vi "glb_data.vi"() -> ()   [LabVIEW 2014]
panel:
  in  "冷却系统模块":T1(array[cluster])
  in  "冷却系统模块值":string[](array[string])
  in  "FPGA模块值":string[](array[string])
  in  "主界面配置类":T2={"侧边栏数据"=[], "界面刷间隔率"=1000.0}
  in  "show配置":T3
  in  "测试模块值8":string[](array[string])
  in  "测试模块值7":string[](array[string])
  in  "测试模块值6":string[](array[string])
  in  "测试模块值5":string[](array[string])
  in  "测试模块值4":string[](array[string])
  in  "测试模块值3":string[](array[string])
  in  "测试模块值2":string[](array[string])
  in  "测试模块值1":string[](array[string])
  in  "cRIO模块值":string[](array[string])
  in  "GPS模块值":string[](array[string])
  in  "OBD模块值":string[](array[string])
  in  "cRIO模块":T1(array[cluster])
  in  "测试模块8":T1(array[cluster])
  in  "测试模块7":T1(array[cluster])
  in  "测试模块6":T1(array[cluster])
  in  "测试模块5":T1(array[cluster])
  in  "测试模块4":T1(array[cluster])
  in  "测试模块3":T1(array[cluster])
  in  "测试模块2":T1(array[cluster])
  in  "测试模块1":T1(array[cluster])
  in  "GPS模块":T1(array[cluster])
  in  "OBD模块":T1(array[cluster])
  in  "数据属性":T4
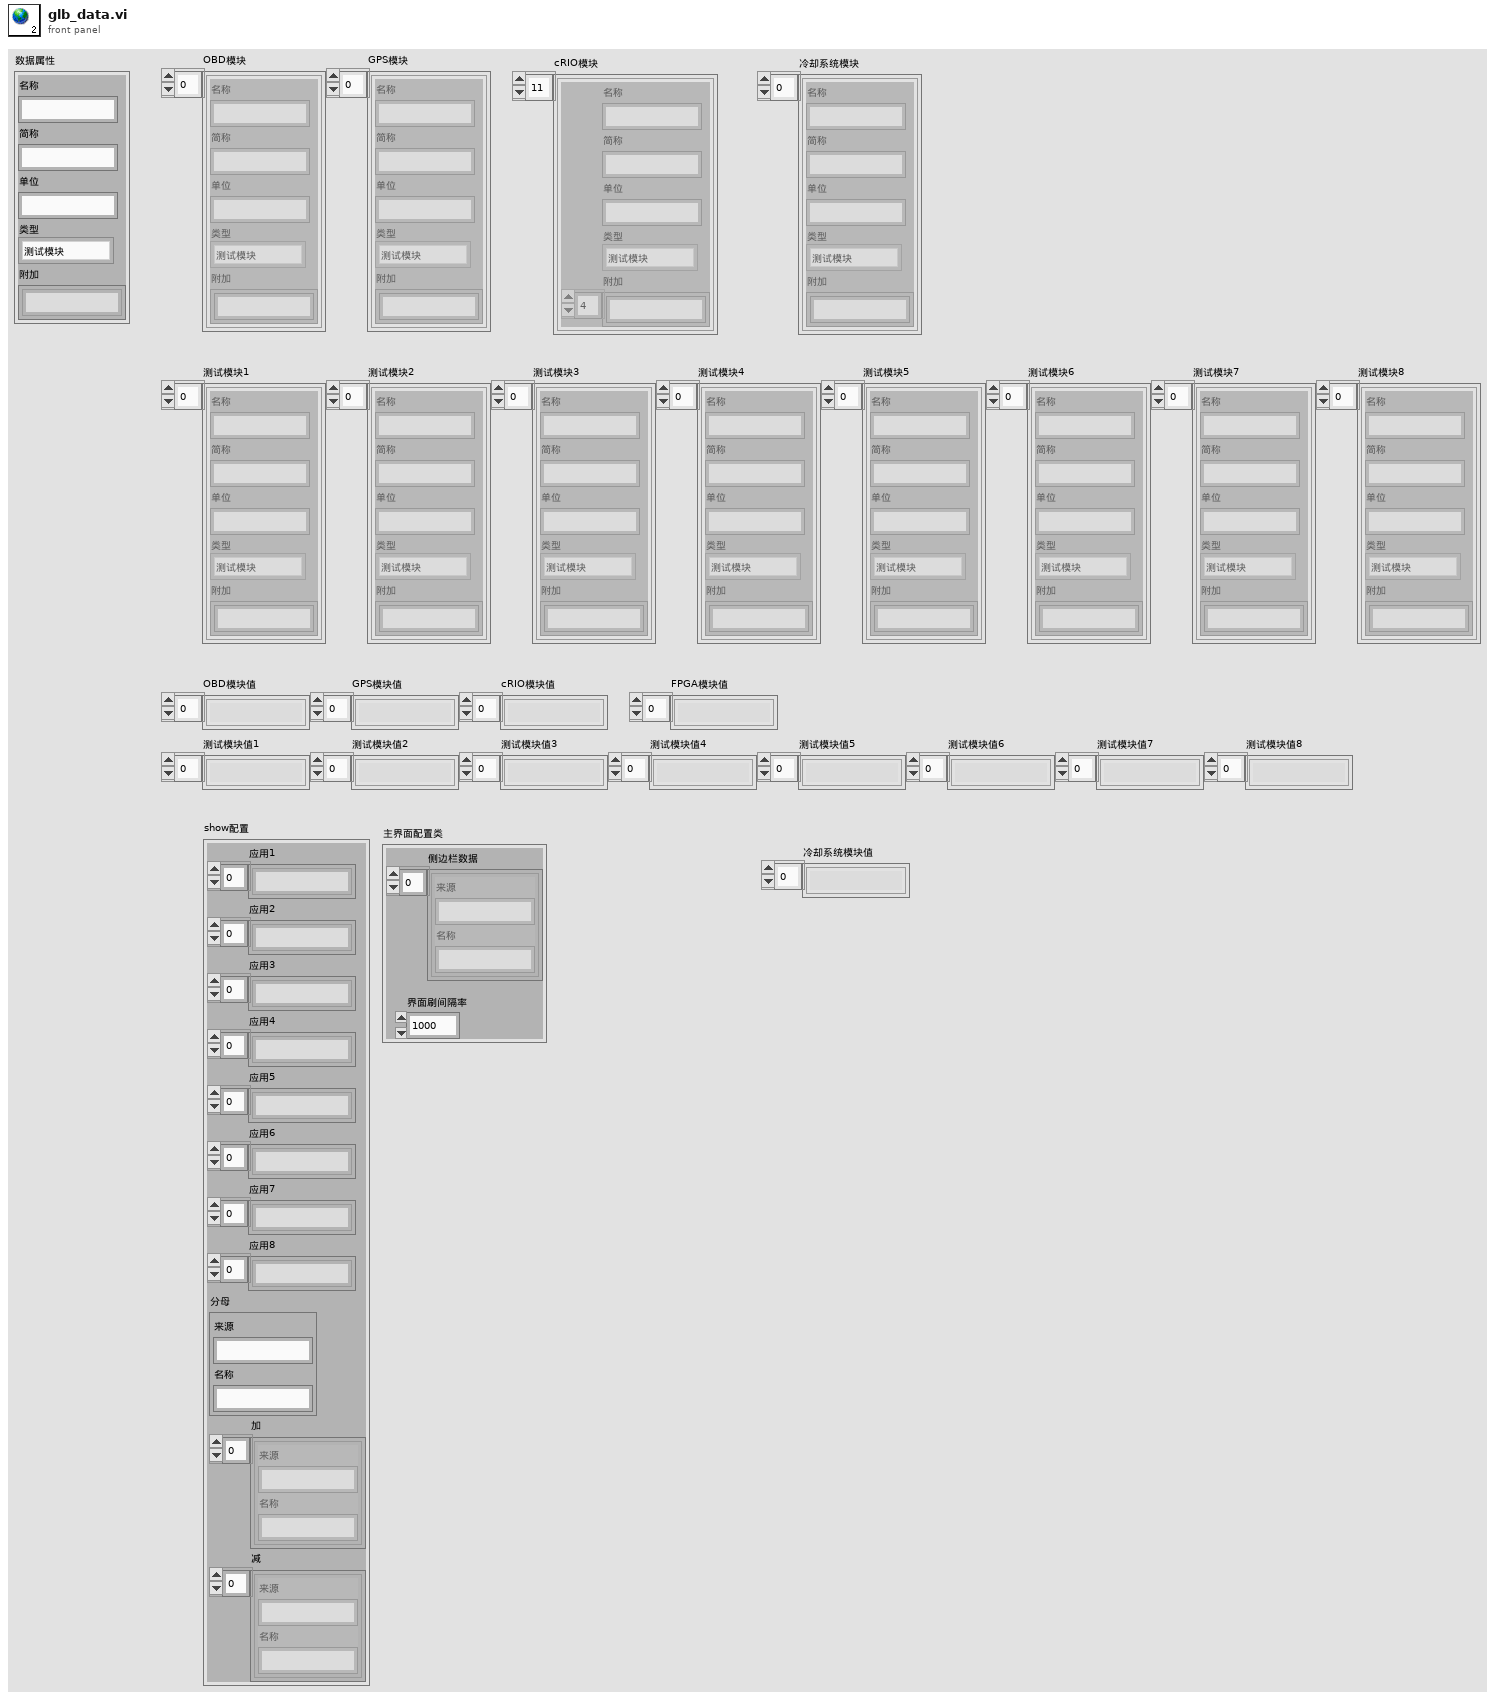
[diagram p1: front panel]
types:
  T1 = cluster{"名称":string, "简称":string, "单位":string, "附加":string[], "类型":enum16{"测试模块", "FPGA", "cRIO", "其他设备", "总体展示"}}[]
  T2 = cluster{"侧边栏数据":cluster{"来源":string, "名称":string}[], "界面刷间隔率":dbl}
  T3 = cluster{"应用1":string[], "应用2":string[], "应用3":string[], "应用4":string[], "应用5":string[], "应用6":string[], "应用7":string[], "应用8":string[], "分母":cluster{"来源":string, "名称":string}, "加":cluster{"来源":string, "名称":string}[], "减":cluster{"来源":string, "名称":string}[]}
  T4 = cluster{"名称":string, "简称":string, "单位":string, "附加":string[], "类型":enum16{"测试模块", "FPGA", "cRIO", "其他设备", "总体展示"}}
diagram:
